vi "Stop Core.vi"(10 "final error code":i32, 11 "CS++StartActor in":refnum<class "CS++StartActor.lvclass">) -> (3 "CS++StartActor out":refnum<class "CS++StartActor.lvclass">)   [LabVIEW 2013, in "CS++StartActor.lvlib" / "CS++StartActor.lvclass"]
doc: "(<B>Filename</B>: Actor Framework.lvlib:Actor.lvclass:Stop Core.vi)\n\nDefines what the actor does before it stops. Use the <B>final error code</B> input to determine whether the actor shut down in response to an error.\n\nBy default, this method does nothing. A descendant class may override it to define behavior, such as shutting down any processes the actor initiated in its override of the Actor Core method."
uses:
  CS++StartActor.lvclass
  CS++BaseActor/CS++BaseActor.lvclass
  CS++StartActor.lvclass/CS++StartActor.ctl
  <vilib>/ActorFramework/Message Enqueuer/Message Enqueuer.lvclass/Message Enqueuer.ctl
  <vilib>/ActorFramework/Message Enqueuer/Enqueue.vi
  <vilib>/ActorFramework/Message Priority Queue/Priority Enqueue.vi
  <vilib>/ActorFramework/Stop Msg/Stop Msg.lvclass
  Libraries/MessageLogger/CS++MessageLogger.lvlib
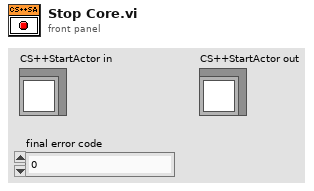
[diagram p1: front panel]
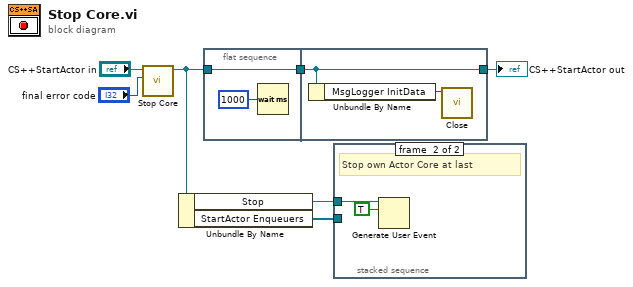
[diagram p0: block diagram]
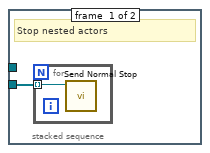
[diagram p2: hidden frame]
diagram:
  n1 = call-parent "Stop Core.vi"("final error code"="final error code", "CS++BaseActor in"="CS++StartActor in") -> ("CS++BaseActor out"=w3:refnum<class "CS++StartActor.lvclass">)  [unwired: 9 in]
  n2 = Unbundle By Name(w3) -> ("Stop"=w2:refnum<user-event>, "StartActor Enqueuers"=w1:refnum<class "Message Enqueuer.lvclass">[])
  n3 = flat-sequence {
    tunnel: w3 -> [w9]
    tunnel: [w9] -> w4
    tunnel: [w11] -> w5
    tunnel: w4 -> [w11]
    frame #0 {
      n4 = Wait (ms)(milliseconds to wait=u32 1000) -> ()  [unwired: 1 out]
    }
    frame #1 {
      n5 = Unbundle By Name(w11) -> ("MsgLogger InitData"=w10:variant)
      n6 = call "Close.vi"("Initialization Data"=w10) -> ()  [unwired: 10 in, 1 out]
    }
  }
  n7 = stacked-sequence {
    tunnel: w2 -> [_ w14]
    tunnel: w1 -> [w12 _]
    frame #0 {
      # "Stop nested actors"
      n8 = for {
        tunnel: w12 -> [w13] mode=indexing
        n9 = call <vilib>:"Send Normal Stop.vi"("Message Enqueuer"=w13) -> ()  [unwired: 10 in, 1 out]
      }
    }
    frame #1 {
      # "Stop own Actor Core at last"
      n10 = Generate User Event(user event=w14, event data cluster=TRUE ("event data")) -> ()  [unwired: 2 in, 2 out]
    }
  }
  "CS++StartActor out" <- w5
